vi "Resize 1D Array.vi"(4 "array size":i32, 5 "input array":dbl[](array[numeric]) format="%.2f") -> (2 "output array":dbl[](array[numeric]) format="%.2f")   [LabVIEW 2012]
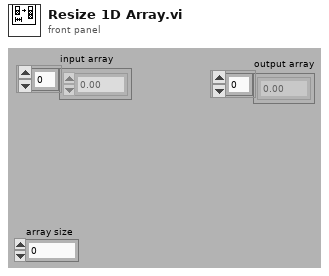
[diagram p1: front panel]
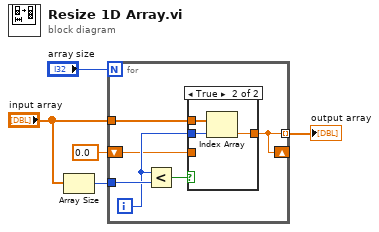
[diagram p0: block diagram]
diagram:
  n1 = Array Size(array="input array") -> (size(s)=w2:i32)
  n2 = for {
    N: "array size" -> [_]
    tunnel: w2 -> [w8]
    tunnel: "input array" -> [w11]
    tunnel: [w10] -> w3 mode=indexing
    shift-right: [w10] -> _
    shift-left: 0.0 ("Numeric") -> [w6]
    i -> [w7]
    n3 = Less?(x=w7, y=w8) -> (x < y?=w9:bool)
    n4 = case shown="True" w9 {
      tunnel: w11 -> [_ w15]
      tunnel: [w12 w14] -> w10
      tunnel: w7 -> [_ w13]
      tunnel: w6 -> [w12 _]
      frame False {
      }
      frame True {
        n5 = Index Array(array=w15, index=w13) -> (element=w14:dbl)
      }
    }
  }
  "output array" <- w3
